vi "Get configuration chain.vi"(8 "error in (no error)":errorcluster, 11 "focusBase in":refnum<class "focus.lvclass">) -> (0 "error out":errorcluster, 1 "class name":string[](array[string]), 2 "configuration chain":variant[](array[variant]), 3 "focusBase out":refnum<class "focus.lvclass">)   [LabVIEW 2012, in "focus.lvclass"]
doc: "Returns an array of variants containing the configuration clusters of each class in the inheritance chain (lowest child class first), together with an array of all class names in the inheritance chain.\n\nFor classes without configuration cluster, the configuration chain contains empty variants."
uses:
  focus.lvclass
  <vilib>/Distrio/Murmex/Murmex/Murmex.lvclass
  focus.lvclass/focus.ctl
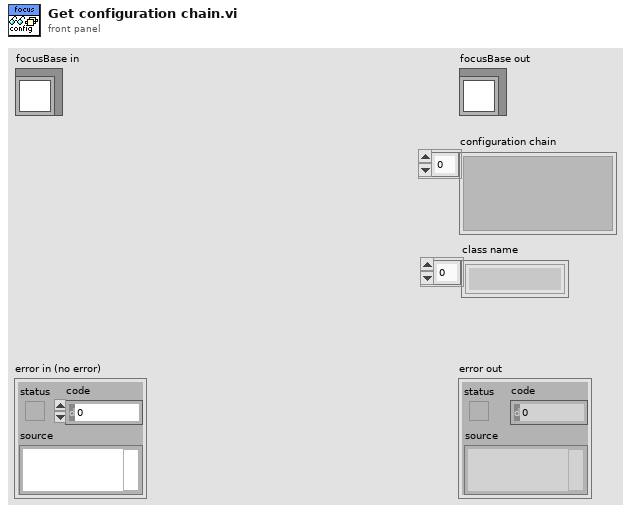
[diagram p1: front panel]
types:
  T1 = typedef "focus.lvclass/configuration_cluster.ctl" = cluster{"Port":T2, "Baudrate":T3, "update frequency":dbl[unit], "S/N Master controller":string, "Interface":T4, "soft limit min":dbl, "soft limit max":dbl, "startup speed":dbl[unit]}
  T2 = typedef "focus.lvclass/port_focus.ctl" = i32
  T3 = typedef "focus.lvclass/baud_rate_focus.ctl" = u16
  T4 = typedef "focus.lvclass/connection_type_focus.ctl" = enum16{"RS232", "RS232 DaisyChain", "USB", "USB_DaisyChain"}
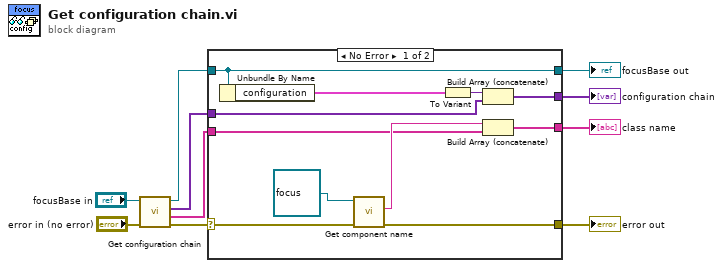
[diagram p0: block diagram]
diagram:
  n1 = call-parent "Get configuration chain.vi"("error in (no error)"="error in (no error)", "MurmexBase in"="focusBase in") -> ("error out"=w8:errorcluster, "class name"=w2:string[], "configuration chain"=w4:variant[], "MurmexBase out"=w6:refnum<class "focus.lvclass">)  [unwired: 6 in]
  n2 = case shown="No Error" w8 {
    selector: w8 -> [w21 w25]
    tunnel: [w19 w25] -> w7
    tunnel: w6 -> [w17 w24]
    tunnel: [w17 w24] -> w5
    tunnel: w4 -> [w15 w23]
    tunnel: [w14 w23] -> w3
    tunnel: w2 -> [w12 w22]
    tunnel: [w11 w22] -> w1
    frame No Error {
      n3 = Unbundle By Name(w17) -> ("configuration"=w16:T1)
      n4 = call <vilib>:"Get component name.vi"("error in (no error)"=w21, "Murmex in"=refnum<class "focus.lvclass"> refnum ("focus")) -> ("error out"=w19:errorcluster, "component name"=w13:string)  [unwired: 7 in, 1 out]
      n5 = To Variant(anything=w16) -> (Variant=w18:variant)
      n6 = Build Array (concatenate)(w18, w15) -> (w14:variant[])
      n7 = Build Array (concatenate)(w13, w12) -> (w11:string[])
    }
    frame Error {
    }
  }
  "error out" <- w7
  "focusBase out" <- w5
  "configuration chain" <- w3
  "class name" <- w1
